vi "Stop by ID.vi"(8 "Module ID":i32, 10 "Module Lib":refnum<vi>, 11 "References Map":map{string, refnum<vi>}(c390)) -> (0 "error out":errorcluster)   [LabVIEW 2020, in "Panter Dashboard.lvlib"]
uses:
  Panter Dashboard.lvlib
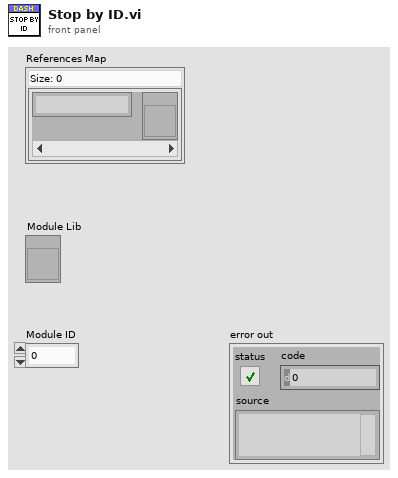
[diagram p1: front panel]
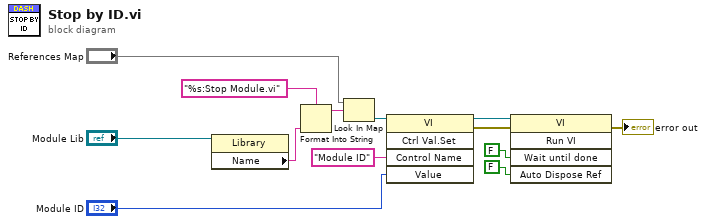
[diagram p0: block diagram]
diagram:
  n1 = property class="Library"(reference="Module Lib") -> ("Name"=w1:string)  [unwired: 1 in, 2 out]
  n2 = Format Into String(format string="%s:Stop Module.vi", w1) -> (resulting string=w8:string)  [unwired: 2 in, 1 out]
  n3 = Look In Map(map="References Map", key=w8) -> (value=w6:refnum<vi>)  [unwired: 1 in, 1 out]
  n4 = invoke class="VI" method="Ctrl Val.Set"(reference=w6, "Control Name"="Module ID", "Value"="Module ID") -> (reference out=w3:refnum<vi>, error out=w12:errorcluster)  [unwired: 2 in, 3 out]
  n5 = invoke class="VI" method="Run VI"(reference=w3, error in=w12, "Wait until done"=FALSE ("Wait Until Done"), "Auto Dispose Ref"=FALSE ("Auto Dispose Reference")) -> (error out=→"error out":errorcluster)  [unwired: 1 in, 4 out]
